vi "Initialize.vi"(8 "error in (no error)":errorcluster, 11 "Zenoh in":refnum<class "Zenoh.lvclass">) -> (0 "error out":errorcluster, 3 "Zenoh out":refnum<class "Zenoh.lvclass">)   [LabVIEW 2021, in "Zenoh.lvclass"]
uses:
  Zenoh.lvclass
  Zenoh.lvclass/Zenoh.ctl
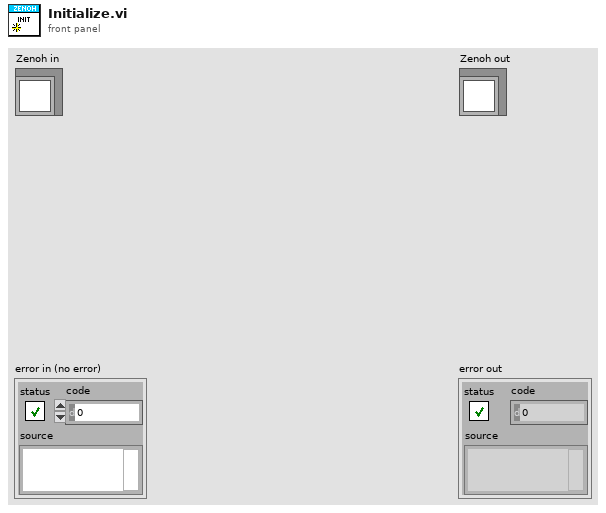
[diagram p1: front panel]
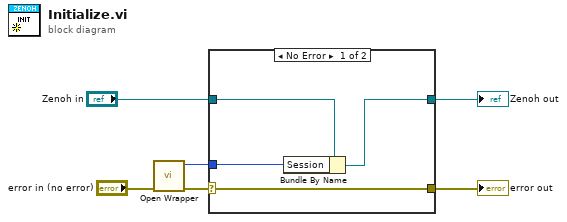
[diagram p0: block diagram]
diagram:
  n1 = call "Open Wrapper.vi"("error in (no error)"="error in (no error)") -> ("error out"=w2:errorcluster, "Session"=w1:i64)  [unwired: 9 in]
  n2 = case shown="No Error" w2 {
    selector: w2 -> [w7 w12]
    tunnel: [w7 w12] -> w6
    tunnel: [w8 w11] -> w4
    tunnel: "Zenoh in" -> [w9 w11]
    tunnel: w1 -> [w10 _]
    frame No Error {
      n3 = Bundle By Name(cluster=w9, "Session"=w10) -> (w8:refnum<class "Zenoh.lvclass">)
    }
    frame Error {
    }
  }
  "error out" <- w6
  "Zenoh out" <- w4
